vi "Start Mavproxy.vi"   [LabVIEW 2014]
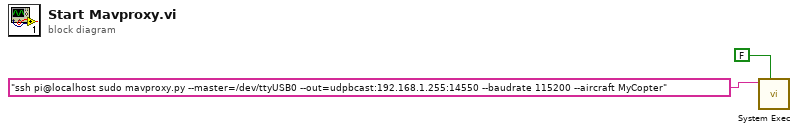
[diagram p0: block diagram]
diagram:
  n1 = call <vilib>:"System Exec.vi"("wait until completion? (T)"=FALSE, "command line"="ssh pi@localhost sudo mavproxy.py --master=/dev/ttyUSB0 --out=udpbcast:192.168.1.255:14550 --baudrate 115200 --aircraft MyCopter") -> ()  [unwired: 6 in, 4 out]
